vi "Initialize Input DMA Refs.vi"(8 "error in (no error)":errorcluster, 10 "Settings.Compiled":T1 {"IncomingRegisters.Settings"."Register"."Data Type" format="%.0x"; "IncomingRegisters.Refs"."Refs"."Data Reference" format="%.0x"; "OutgoingRegisters.Settings"."Register"."Data Type" format="%.0x"; "OutgoingRegisters.Refs"."Refs"."Data Reference" format="%.0x"; "IncomingDMA.Settings"."DMA.Settings"."dt" format="%#_p"; "IncomingDMA.Settings"."DMA.Settings"."Update Rate" items=["1 Hz"=1, "2 Hz"=2, "5 Hz"=5, "10 Hz"=10]; "IncomingDMA.Settings"."WritetoVSEngine.Refs"."Refs" format="%.0x"; "OutgoingDMA.Settings"."DMA.Settings"."dt" format="%#_p"; "OutgoingDMA.Settings"."DMA.Settings"."Update Rate" items=["1 Hz"=1, "2 Hz"=2, "5 Hz"=5, "10 Hz"=10]; "OutgoingDMA.Settings"."WritetoVSEngine.Refs"."Refs" format="%.0x"}, 11 "FPGA Ref":refnum<k20>) -> (0 "error out":errorcluster, 2 "DMA Settings":T14[](array[typedef]) {"DMA Settings"."dt" format="%#_p"; "DMA Settings"."Update Rate" items=["1 Hz"=1, "2 Hz"=2, "5 Hz"=5, "10 Hz"=10]; "Write to VS Engine.Refs"."Refs" format="%.0x"}, 3 "FPGA Ref":refnum<k20>)   [LabVIEW 2015, in "FPGA Addon Engine.lvlib"]
uses:
  FPGA Addon Engine.lvlib
  Types/DMA Input References.ctl
  <vilib>/NI Veristand/Custom Device Waveform API/Multiple Waveforms Write (DBL)/Multiple Waveforms Write (DBL).lvclass
  Types/DMA Input Ref.ctl
  <vilib>/NI Veristand/Custom Device API/Data Reference.ctl
  Shared/DMA Settings.ctl
  Shared/Delacing Scheme.ctl
  Shared/DMA Acquisition Mode.ctl
  Shared/Compiled.Settings
  Shared/Compiled.RegisterSettings.ctl
  Shared/Scalar Type.ctl
  Shared/Register Information.ctl
  <userlib>/_OpenG.lib/lvdata/lvdata.llb/Type Descriptor Enumeration__ogtk.ctl
  <vilib>/NI Veristand/Custom Device API/Block Data Reference.ctl
  Shared/Compiled.DMASettings.ctl
  <vilib>/NI Veristand/Custom Device API/Waveform Data Reference.ctl
  Shared/FPGA Settings.ctl
  <vilib>/NI/LVFPGA Adv Session Resources/OpenByNameSubVI.vi
  <vilib>/NI Veristand/Custom Device Waveform API/Multiple Waveforms Write (DBL)/NI VeriStand - Open Multiple Waveforms Write Session (DBL).vi
  <vilib>/Utility/error.llb/Error Cluster From Error Code.vi
  <vilib>/rvi/interface/common/niFpgaWaitOnOcc.vi
  <vilib>/rvi/interface/common/dynamic/niFpgaEscapeDelimiterAndNull.vi
  <vilib>/rvi/interface/nirviMethod/nirviMethod.xnode
  <vilib>/NI/LVFPGA Adv Session Resources/OpenByName.xnode
  <vilib>/NI VeriStand/Custom Device Waveform API/NI_VS Custom Device Waveform API.lvlib
  <vilib>/rvi/errors/niLvFpgaMergeErrorWithErrorCode.vi
  <vilib>/NI VeriStand/Custom Device API/Custom Device API.lvlib
  Shared/FPGA Addon Shared.lvlib
  <vilib>/FPGAPlugInAG/Dynamic/niLvFpga_ConfigureFifo_Dynamic.vi
  <vilib>/FPGAPlugInAG/Dynamic/niLvFpga_StartFifo_Dynamic.vi
  <vilib>/NI/LVFPGA Adv Session Resources/LVFPGAAdvSessionResources.lvlib
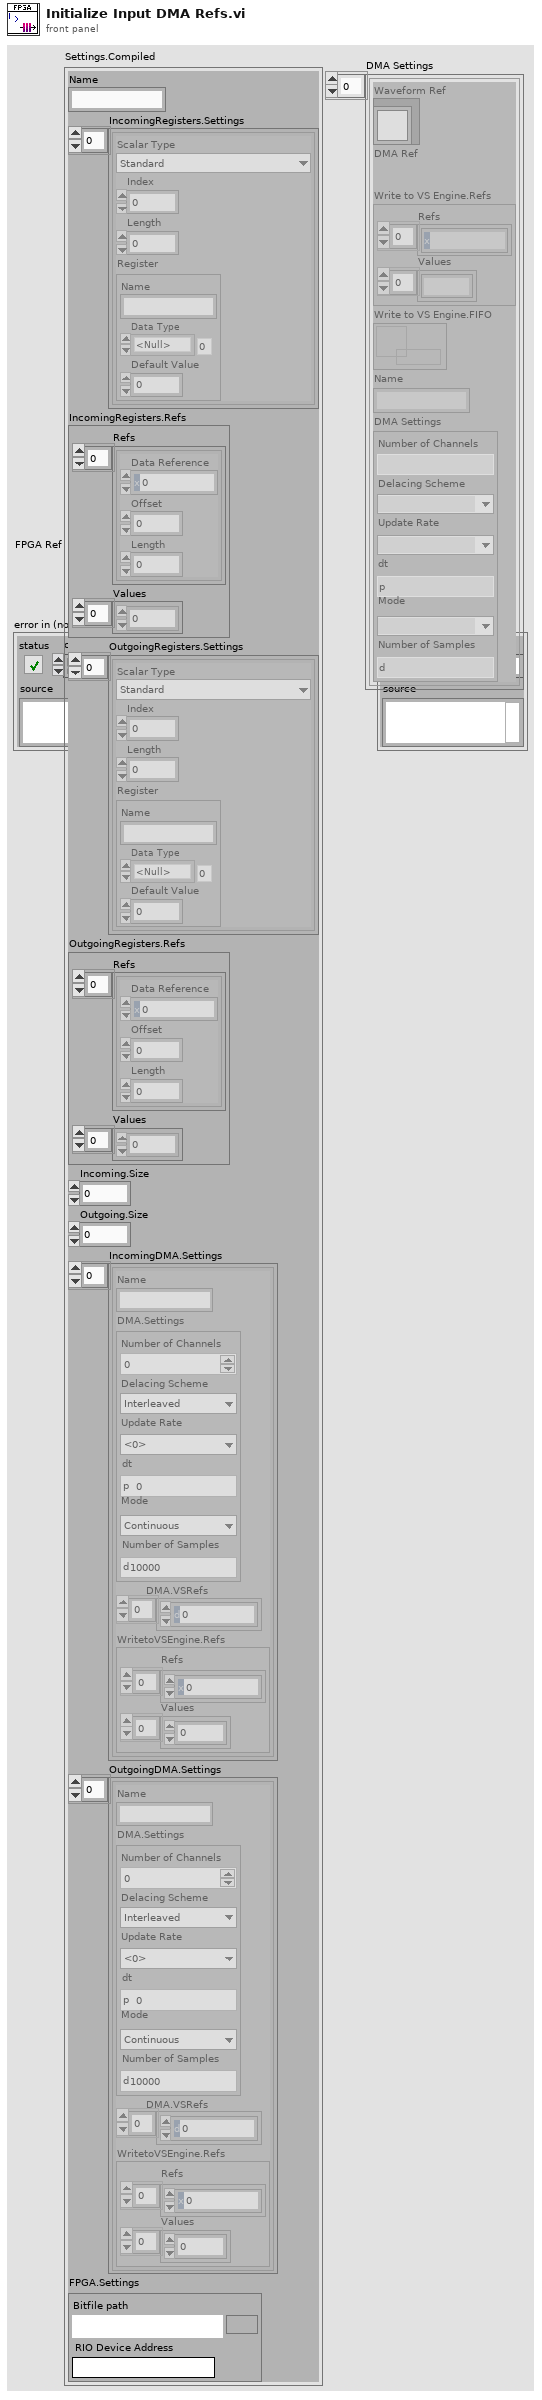
[diagram p1: front panel]
types:
  T1 = typedef "FPGA Addon Shared.lvlib/Compiled.Settings" = cluster{"Name":string, "IncomingRegisters.Settings":T2[], "IncomingRegisters.Refs":cluster{"Refs":T6[], "Values":dbl[]}, "OutgoingRegisters.Settings":T2[], "OutgoingRegisters.Refs":cluster{"Refs":T6[], "Values":dbl[]}, "Incoming.Size":i32, "Outgoing.Size":i32, "IncomingDMA.Settings":T8[], "OutgoingDMA.Settings":T8[], "FPGA.Settings":T13}
  T2 = typedef "FPGA Addon Shared.lvlib/Compiled.RegisterSettings.ctl" = cluster{"Scalar Type":T3, "Index":i32, "Length":i32, "Register":T4}
  T3 = typedef "FPGA Addon Shared.lvlib/Scalar Type.ctl" = enum16{"Standard", "Bitpacked"}
  T4 = typedef "FPGA Addon Shared.lvlib/Register Information.ctl" = cluster{"Name":string, "Data Type":T5, "Default Value":dbl}
  T5 = typedef "Type Descriptor Enumeration__ogtk.ctl" = enum8{"<Null>", "I8", "I16", "I32", "I64", "U8", "U16", "U32", "U64", "SGL", "DBL", "EXT", "CSG", "CDB", "CXT", "0x0F", "0x10", "0x11", "0x12", "0x13", "0x14", "Enum U8", "Enum U16", "Enum U32", "Enum U64", "SGL PQ", "DBL PQ", "EXT PQ", "CSG PQ", "CDB PQ", "CXT PQ", "0x1F", "0x20", "Boolean", "0x22", "0x23", "0x24", "0x25", "0x26", "0x27", "0x28", "0x29", "0x2A", "0x2B", "0x2C", "0x2D", "0x2E", "0x2F", "String", "0x31", "Path", "Pict", "0x34", "0x35", "0x36", "DAQ", "0x38", "0x39", "0x3A", "0x3B", "0x3C", "0x3D", "0x3E", "0x3F", "Array", "0x41", "0x42", "0x43", "0x44", "0x45", "0x46", "0x47", "0x48", "0x49", "0x4A", "0x4B", "0x4C", "0x4D", "0x4E", "0x4F", "Cluster", "0x51", "0x52", "Variant", "Waveform", "0x55", "0x56", "0x57", "0x58", "0x59", "0x5A", "0x5B", "0x5C", "0x5D", "0x5E", "0x5F", "0x60", "0x61", "0x62", "0x63", "0x64", "0x65", "0x66", "0x67", "0x68", "0x69", "0x6A", "0x6B", "0x6C", "0x6D", "0x6E", "0x6F", "Refnum"}
  T6 = typedef "Custom Device API.lvlib/Block Data Reference.ctl" = cluster{"Data Reference":T7, "Offset":u64, "Length":u64}
  T7 = typedef "Custom Device API.lvlib/Data Reference.ctl" = i32
  T8 = typedef "FPGA Addon Shared.lvlib/Compiled.DMASettings.ctl" = cluster{"Name":string, "DMA.Settings":T9, "DMA.VSRefs":T12[], "WritetoVSEngine.Refs":cluster{"Refs":T7[], "Values":dbl[]}}
  T9 = typedef "FPGA Addon Shared.lvlib/DMA Settings.ctl" = cluster{"Number of Channels":u8, "Delacing Scheme":T10, "Update Rate":u32, "dt":dbl, "Mode":T11, "Number of Samples":u32}
  T10 = typedef "FPGA Addon Shared.lvlib/Delacing Scheme.ctl" = enum8{"Interleaved"}
  T11 = typedef "FPGA Addon Shared.lvlib/DMA Acquisition Mode.ctl" = enum8{"Continuous", "Triggered Finite"}
  T12 = typedef "Custom Device API.lvlib/Waveform Data Reference.ctl" = i32
  T13 = typedef "FPGA Addon Shared.lvlib/FPGA Settings.ctl" = cluster{"Bitfile path":path, "RIO Device Address":string}
  T14 = typedef "FPGA Addon Engine.lvlib/DMA Input References.ctl" = cluster{"Waveform Ref":refnum<class "Multiple Waveforms Write (DBL).lvclass">, "DMA Ref":T15, "Write to VS Engine.Refs":cluster{"Refs":T7[], "Values":dbl[]}, "Write to VS Engine.FIFO":refnum<k33>, "Name":string, "DMA Settings":T9}
  T15 = typedef "FPGA Addon Engine.lvlib/DMA Input Ref.ctl" = refnum<k20>
  T16 = cluster{"read mode":enum16{"polling", "blocking"}, "write mode":enum16{"polling", "blocking"}}
  T17 = cluster{"Name":string, "Depth":u32, "Write? (Deprecated:Use Implementation)":bool, "Physical Channel":u32, "Base Address":u32, "Data Width":u32, "Data Type":enum32{"Boolean", "I8", "I16", "I32", "I64", "U8", "U16", "U32", "U64", "FXP", "CustomControl", "SGL"}, "FXP Properties":variant, "Write Window Address":u32, "Implementation":enum16{"niFpgaTargetToHost", "niFpgaHostToTarget", "niFpgaPeerToPeerWriter", "niFpgaPeerToPeerReader", "niCoreTargetToHost", "niCoreHostToTarget"}, "Control Set":u32}[]
  T18 = cluster{"Name":string, "type":variant, "indicator?":bool}[]
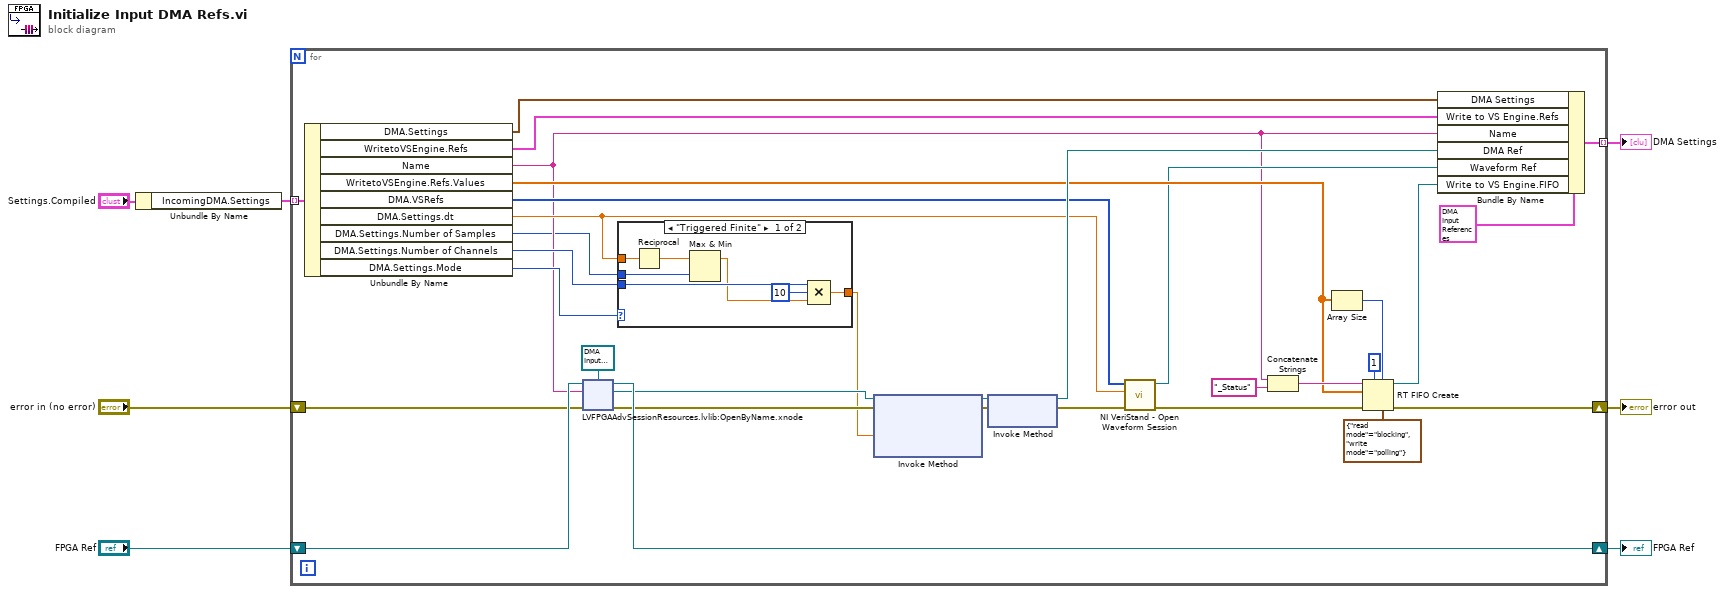
[diagram p0: block diagram]
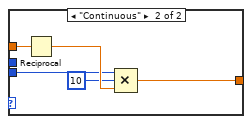
[diagram p2: hidden frame]
diagram:
  n1 = Unbundle By Name("Settings.Compiled") -> ("IncomingDMA.Settings"=w3:T8[])
  n2 = for {
    shift-right: [w37] -> w6
    shift-left: "FPGA Ref" -> [w38]
    tunnel: [w36] -> w5 mode=indexing
    tunnel: w3 -> [w27] mode=indexing
    shift-right: [w16] -> w2
    shift-left: "error in (no error)" -> [w22]
    n3 = Unbundle By Name(w27) -> ("DMA.Settings"=w14:T9, "WritetoVSEngine.Refs"=w25:cluster{"Refs":T7[], "Values":dbl[]}, "Name"=w9:string, "WritetoVSEngine.Refs.Values"=w20:dbl[], "DMA.VSRefs"=w21:T12[], "DMA.Settings.dt"=w28:dbl, "DMA.Settings.Number of Samples"=w8:u32, "DMA.Settings.Number of Channels"=w17:u8, "DMA.Settings.Mode"=w10:T11)
    n4 = xnode "LVFPGAAdvSessionResources.lvlib:OpenByName.xnode"("FPGA VI Reference in"=w38, "Resource name in"=w9, "Single resource reference type in"=T15 refnum, "Error in"=w22) -> ("Single resource reference out"=w32:T15, "Error out"=w33:errorcluster, "FPGA VI Reference out"=w37:refnum<k20>)
    n5 = case shown="\"Triggered Finite\"" w10 {
      tunnel: [w44 w49] -> w29
      tunnel: w28 -> [w43 w48]
      tunnel: w17 -> [w45 w47]
      tunnel: w8 -> [w41 _]
      frame "Triggered Finite" {
        n6 = Reciprocal(x=w43) -> (1/x=w42:dbl)
        n7 = Max & Min(x=w42, y=w41) -> (max(x,y)=w40:dbl)  [unwired: 1 out]
        n8 = Compound Arithmetic op=MULTIPLY(w45, u8 10 ("value"), w40) -> (w44:dbl)
      }
      frame "Continuous" {
        n9 = Reciprocal(x=w48) -> (1/x=w51:dbl)
        n10 = Compound Arithmetic op=MULTIPLY(w47, u8 10 ("value"), w51) -> (w49:dbl)
      }
    }
    n11 = xnode "Invoke Method"("FPGA VI Reference In"=w32, "error in"=w33, "Requested Depth"=w29) -> ("FPGA VI Reference Out"=w35:T15, "error out"=w34:errorcluster)  [unwired: 1 out]
    n12 = xnode "Invoke Method"("FPGA VI Reference In"=w35, "error in"=w34) -> ("FPGA VI Reference Out"=w31:T15, "error out"=w24:errorcluster)
    n13 = call-poly <vilib>:"NI VeriStand - Open Waveform Session.vi"("error in (no error)"=w24, "dt"=w28, "DBL Waveform Data References"=w21) -> ("error out"=w23:errorcluster, "Multiple Waveforms Write Session (DBL)"=w18:refnum<class "Multiple Waveforms Write (DBL).lvclass">)  [unwired: 7 in]
    n14 = Concatenate Strings(w9, "_Status" ("FIFO Name")) -> (w26:string)
    n15 = Array Size(array=w20) -> (size(s)=w13:i32)
    n16 = RT FIFO Create(0:w26, 1:w20, 3:w23, 4:u32 1 ("elements in array (1)"), 6:w13, 7:T16 {"read mode"=enum."blocking", "write mode"=enum."polling"} ("r/w modes (polling,polling)")) -> (8:w19:refnum<k33>, 11:w16:errorcluster)  [unwired: 2 in, 1 out]
    n17 = Bundle By Name(cluster=T14 {"Waveform Ref"=refnum, "DMA Ref"=refnum, "Write to VS Engine.Refs"={"Refs"=[], "Values"=[]}, "Write to VS Engine.FIFO"=refnum, "Name"="", "DMA Settings"={"Number of Channels"=0, "Delacing Scheme"=enum."Interleaved", "Update Rate"=0, "dt"=0.0, "Mode"=enum."Continuous", "Number of Samples"=10000}}, "DMA Settings"=w14, "Write to VS Engine.Refs"=w25, "Name"=w9, "DMA Ref"=w31, "Waveform Ref"=w18, "Write to VS Engine.FIFO"=w19) -> (w36:T14)
  }
  "error out" <- w2
  "FPGA Ref" <- w6
  "DMA Settings" <- w5
